vi "checkTestActive.vi"(8 "error in (no error)":errorcluster, 11 "Model in":refnum<class "Model.lvclass">) -> (0 "error out":errorcluster, 2 "testActiveIsTrue":bool, 3 "Model out":refnum<class "Model.lvclass">)   [LabVIEW 2013, in "Model.lvclass"]
uses:
  Model.lvclass
  Model.lvclass/Model.ctl
  ApplicationElements/TestMonitor/TestMonitor.lvclass/TestMonitor.ctl
  ApplicationElements/TestMonitor/TestMonitor.lvclass
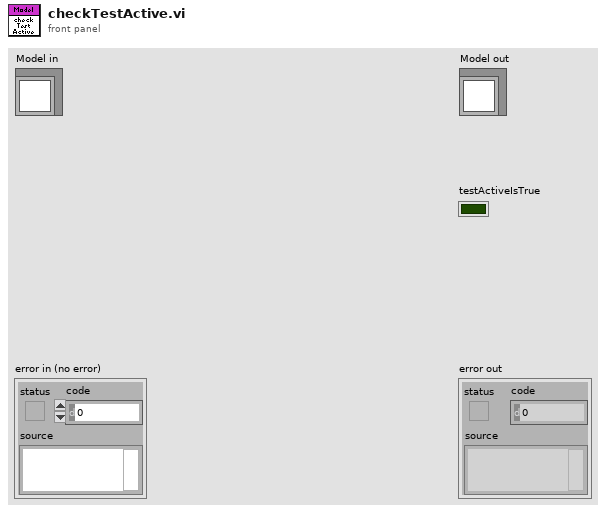
[diagram p1: front panel]
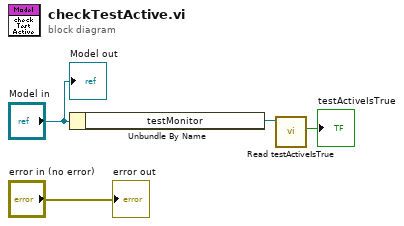
[diagram p0: block diagram]
diagram:
  n1 = Unbundle By Name("Model in") -> ("testMonitor"=w2:refnum<class "TestMonitor.lvclass">)
  n2 = call "Read testActiveIsTrue.vi"("TestMonitor in"=w2) -> ("testActiveIsTrue"=→"testActiveIsTrue":bool)  [unwired: 9 in, 1 out]
  "error out" <- "error in (no error)"
  "Model out" <- "Model in"
